vi "GetInstance.vi"(8 "error in (no error)":errorcluster, 11 "National Instruments USB-8473 Adapter Class in":refnum<class "National Instruments USB-8473 Adapter Class.lvclass">) -> (0 "error out":errorcluster, 2 "Values":string[](array[string]), 3 "National Instruments USB-8473 Adapter Class out":refnum<class "National Instruments USB-8473 Adapter Class.lvclass">)   [LabVIEW 2011, in "National Instruments USB-8473 Adapter Class.lvclass"]
uses:
  National Instruments USB-8473 Adapter Class.lvclass
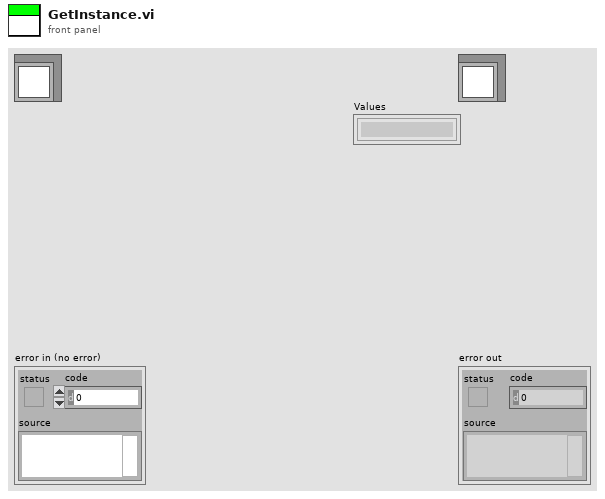
[diagram p1: front panel]
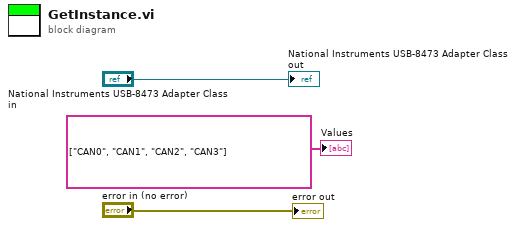
[diagram p0: block diagram]
diagram:
  "error out" <- "error in (no error)"
  "National Instruments USB-8473 Adapter Class out" <- "National Instruments USB-8473 Adapter Class in"
  "Values" <- string[] ["CAN0", "CAN1", "CAN2", "CAN3"] ("Values")
